vi "lvssh2_session_callback_register_receive_32.vi"(11 "receive":refnum<vi>) -> (0 "error out":errorcluster, 2 "stop event":refnum<user-event>, 3 "user event":refnum<user-event>)   [LabVIEW 2017, in "libssh2.lvlib"]
uses:
  libssh2.lvlib
  lvssh2_session_callback_receive_function_input_args_32.ctl
  lvssh2_session_callback_receive_handler_32.vi
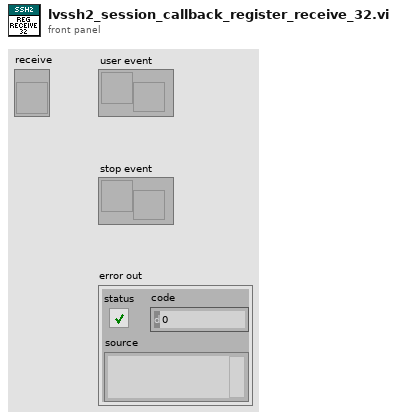
[diagram p1: front panel]
types:
  T1 = typedef "libssh2.lvlib/lvssh2_session_callback_receive_function_input_args_32.ctl" = cluster{"*socket":u32, "*buffer":u32, "length":u32, "flags":i32, "*bytes_received":u32, "completion":u32}
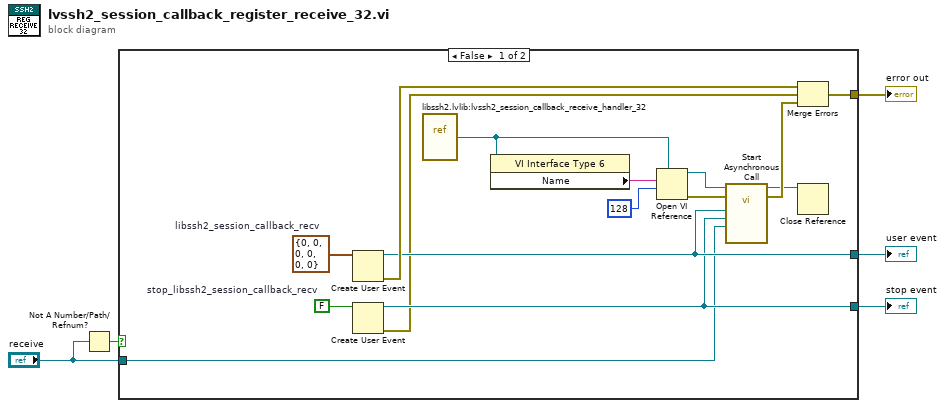
[diagram p0: block diagram]
diagram:
  n1 = Not A Number/Path/Refnum?(number/path/refnum="receive") -> (NaN/Path/Refnum?=w3:bool)
  n2 = case shown="False" w3 {
    tunnel: [w11 _] -> w5
    tunnel: [w20 _] -> w4
    tunnel: "receive" -> [w9 _]
    tunnel: [w10 _] -> w1
    frame False {
      w12 = FALSE  # stop_libssh2_session_callback_recv
      w19 = T1 {"*socket"=0, "*buffer"=0, "length"=0, "flags"=0, "*bytes_received"=0, "completion"=0}  # libssh2_session_callback_recv
      n3 = Create User Event(user event datatype=w19) -> (user event=w11:refnum<user-event>, error out=w18:errorcluster)  [unwired: 1 in]
      n4 = Create User Event(user event datatype=w12) -> (user event=w10:refnum<user-event>, error out=w8:errorcluster)  [unwired: 1 in]
      n5 = vi-ref "libssh2.lvlib:lvssh2_session_callback_receive_handler_32.vi"() -> ("vi reference"=w17:refnum<vi>)
      n6 = property class="VI Interface Type 6"(reference=w17) -> ("Name"=w14:string)  [unwired: 1 in, 2 out]
      n7 = Open VI Reference(type specifier VI Refnum (for type only)=w17, vi path=w14, options=128) -> (vi reference=w16:refnum<vi>, error out=w15:errorcluster)  [unwired: 3 in]
      n8 = call-by-ref "Start Asynchronous Call"(reference=w16, error in=w15, "lvssh2_session_callback_receive"=w9, "Stop Event Ref"=w10, "User Event Ref"=w11) -> (reference out=w6:refnum<vi>, error out=w7:errorcluster)  [unwired: 9 in]
      n9 = Merge Errors(w18, w8, w7) -> (w20:errorcluster)
      n10 = Close Reference(reference=w6) -> ()  [unwired: 1 in, 1 out]
    }
    frame True {
    }
  }
  "user event" <- w5
  "error out" <- w4
  "stop event" <- w1
